vi "Execute.vi"(8 "error in (no error)":errorcluster, 10 ".NET:CheckPqmNtrsAndProductSerialDateService.PqmNtrsAndProductSerialRequest":T1, 11 "CheckPqmNtrsAndProductSerialDateService refnum":refnum<k24>) -> (0 "error out":errorcluster, 2 ".NET:CheckPqmNtrsAndProductSerialDateService.CommonResponse":T2, 3 "CheckPqmNtrsAndProductSerialDateService refnum out":refnum<k24>)   [LabVIEW 2023, in "CheckPqmNtrsAndProductSerialDateService.lvlib"]
uses:
  <userlib>/WebService/_CheckPqmNtrsAndProductSerialDateService/CheckPqmNtrsAndProductSerialDateService.lvlib
  <userlib>/WebService/_CheckPqmNtrsAndProductSerialDateService/CheckPqmNtrsAndProductSerialDateService.dll
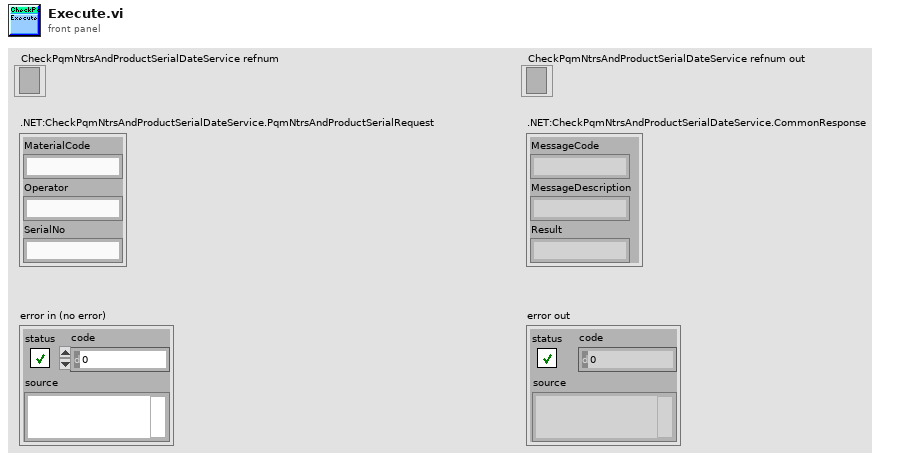
[diagram p1: front panel]
types:
  T1 = cluster{"MaterialCode":string, "Operator":string, "SerialNo":string}
  T2 = cluster{"MessageCode":string, "MessageDescription":string, "Result":string}
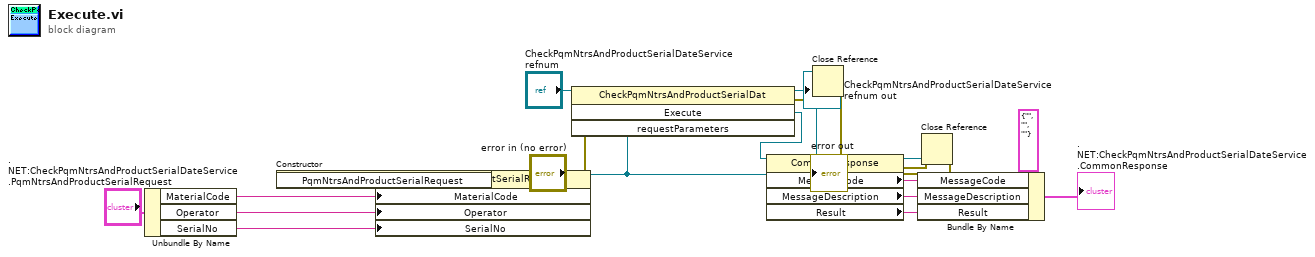
[diagram p0: block diagram]
diagram:
  n1 = Unbundle By Name(".NET:CheckPqmNtrsAndProductSerialDateService.PqmNtrsAndProductSerialRequest") -> ("MaterialCode"=w10:string, "Operator"=w9:string, "SerialNo"=w8:string)
  n2 = constructor class="PqmNtrsAndProductSerialRequest"(error in="error in (no error)") -> (reference out=w14:refnum<k24>, error out=w13:errorcluster)  [unwired: 2 in, 1 out]
  n3 = property class="PqmNtrsAndProductSerialRequest"(reference=w14, error in=w13, "MaterialCode"=w10, "Operator"=w9, "SerialNo"=w8) -> (reference out=w12:refnum<k24>, error out=w6:errorcluster)
  n4 = invoke class="CheckPqmNtrsAndProductSerialDat" method="Execute"(reference="CheckPqmNtrsAndProductSerialDateService refnum", error in=w6, "requestParameters"=w12) -> (reference out=→"CheckPqmNtrsAndProductSerialDateService refnum out":refnum<k24>, error out=w5:errorcluster, "Execute"=w20:refnum<k24>)  [unwired: 1 in, 1 out]
  n5 = Close Reference(reference=w12, error in (no error)=w5) -> (error out=w4:errorcluster)
  n6 = property class="CommonResponse"(reference=w20, error in=w4) -> (reference out=w3:refnum<k24>, error out=w2:errorcluster, "MessageCode"=w17:string, "MessageDescription"=w16:string, "Result"=w15:string)
  n7 = Bundle By Name(cluster=T2 {"MessageCode"="", "MessageDescription"="", "Result"=""} (".NET:CheckPqmNtrsAndProductSerialDateService.CommonResponse"), "MessageCode"=w17, "MessageDescription"=w16, "Result"=w15) -> (→".NET:CheckPqmNtrsAndProductSerialDateService.CommonResponse":T2)
  n8 = Close Reference(reference=w3, error in (no error)=w2) -> (error out=→"error out":errorcluster)
